vi "DAQmx Read (Analog Wfm 1Chan NSamp Duration).vi"(0 "task/channels in":refnum<k21>, 7 "duration":dbl=1.0, 9 "timeout":dbl=10.0 format="%0.2f", 11 "error in":errorcluster) -> (4 "task out":refnum<k21>, 6 "data":waveform(dbl), 15 "error out":errorcluster)   [LabVIEW 2022 SP3]
uses:
  nilvaiu.dll
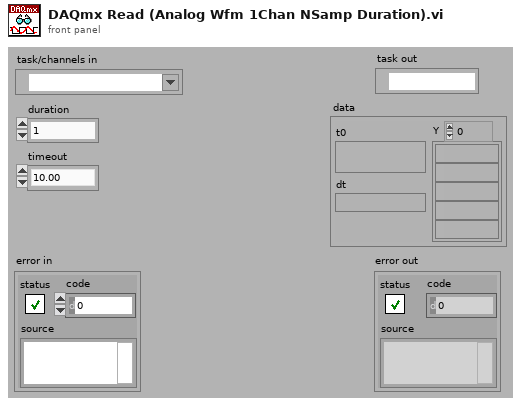
[diagram p1: front panel]
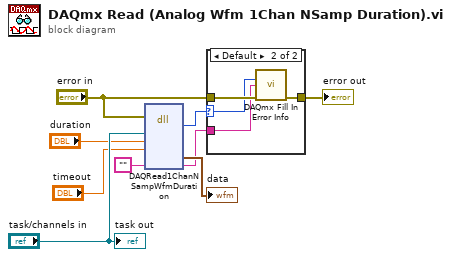
[diagram p0: block diagram]
diagram:
  n1 = dll-call lib="nilvaiu.*" fn="DAQRead1ChanNSampWfmDuration"(error in="error in", "taskID"="task/channels in", "duration"="duration", "timeout"="timeout", "extendedErrorInfo"="") -> ("return type"=w4:i32, "data"=→"data":waveform(dbl), "extendedErrorInfo"=w2:string)  [unwired: 4 in, 4 out]
  n2 = case shown="Default" w4 {
    selector: w4 -> [_ w12]
    tunnel: "error in" -> [w10 w14]
    tunnel: [w10 w13] -> w9
    tunnel: w2 -> [_ w11]
    frame 0 {
    }
    frame Default {
      n3 = call "DAQmx Fill In Error Info.vi"("status code"=w12, "extended error info"=w11, "error in"=w14) -> ("error out"=w13:errorcluster)  [unwired: 1 in, 11 out]
    }
  }
  "error out" <- w9
  "task out" <- "task/channels in"
